vi "Line Configuration Dialog.vi"(8 "error in":errorcluster, 9 "engine configuration in":refnum<class "engine configuration.lvclass">, 10 "TDMS datalogger configuration":refnum<class "TDMS datalogger configuration.lvclass">, 11 "Line":T2) -> (0 "error out":errorcluster, 1 "success":bool, 2 "changed":bool, 3 "Mappings out":T1)   [LabVIEW 2015, in "TDMS datalogger editor node.lvclass"]
uses:
  TDMS datalogger editor node.lvclass
  <vilib>/NI/Module Execution Interface/Engine Configuration/engine configuration.lvclass
  <vilib>/NI/Tag Bus Module Framework/channel/TBM channel.lvclass
  module/configuration/TDMS datalogger configuration.lvclass
  <vilib>/NI/Tag Bus/tag/tag descriptor.lvclass/tag descriptor.ctl
  <vilib>/NI/Configuration Framework/serializable configuration/NISE_CEF_serializable configuration.lvclass/NISE_CEF_serializable configuration.ctl
  <vilib>/NI/Tag Bus/tag/write tag name.vi
  <vilib>/NI/Configuration Framework/serializable configuration/Read UID.vi
  <vilib>/NI/Tag Bus/tag/read data type.vi
  <vilib>/Utility/LVClass/Get LV Class Name.vi
  <vilib>/NI/Configuration Framework/error generator/NISE_error generator.vi
  <vilib>/NI/Tag Bus/tag/tag descriptor.lvclass
  <vilib>/NI/DCAF UI Toolkit/Controls/DCAF UI Elements.lvlib
panel:
  in  "Tag":i32(listbox)
  in  "Property Name":string
  in  "ok":bool
  in  "cancel":bool
  out "errors":string
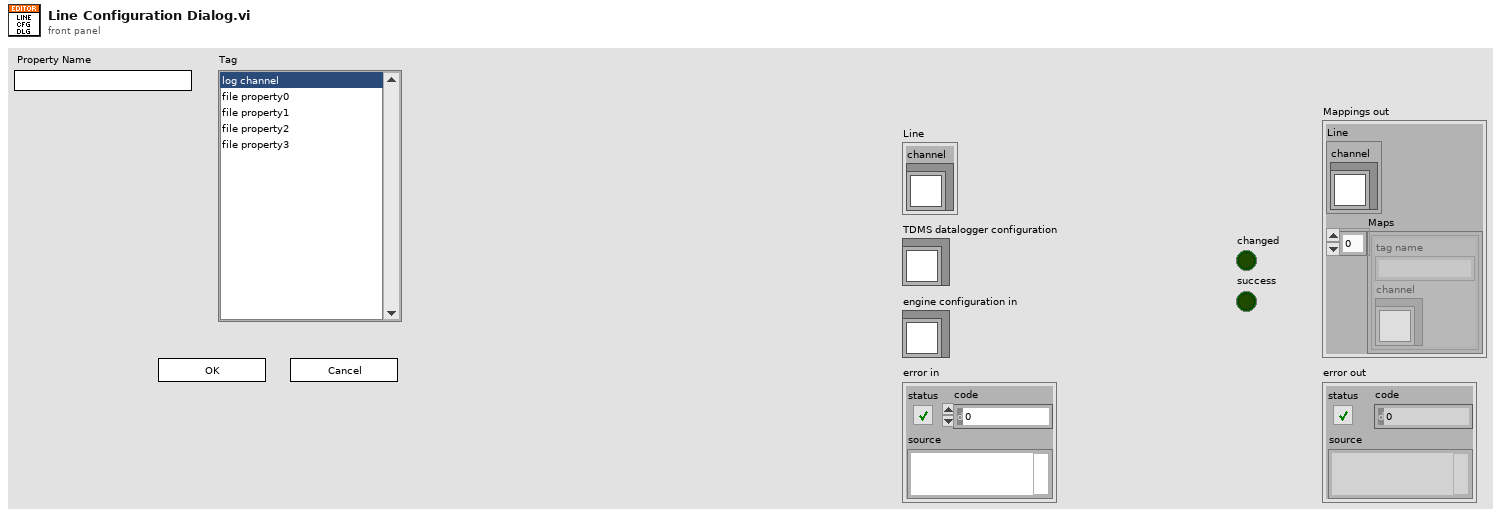
[diagram p1: front panel]
types:
  T1 = cluster{"Line":cluster{"channel":refnum<class "TBM channel.lvclass">}, "Maps":cluster{"tag name":string, "channel":refnum<class "TBM channel.lvclass">}[]}
  T2 = cluster{"channel":refnum<class "TBM channel.lvclass">}
  T3 = enum8{"Enabled", "Disabled", "Disabled and Grayed Out"}
  T4 = cluster{"tag name":string, "channel":refnum<class "TBM channel.lvclass">}
  T5 = cluster{"tag name":string, "channel":refnum<class "TBM channel.lvclass">}[]
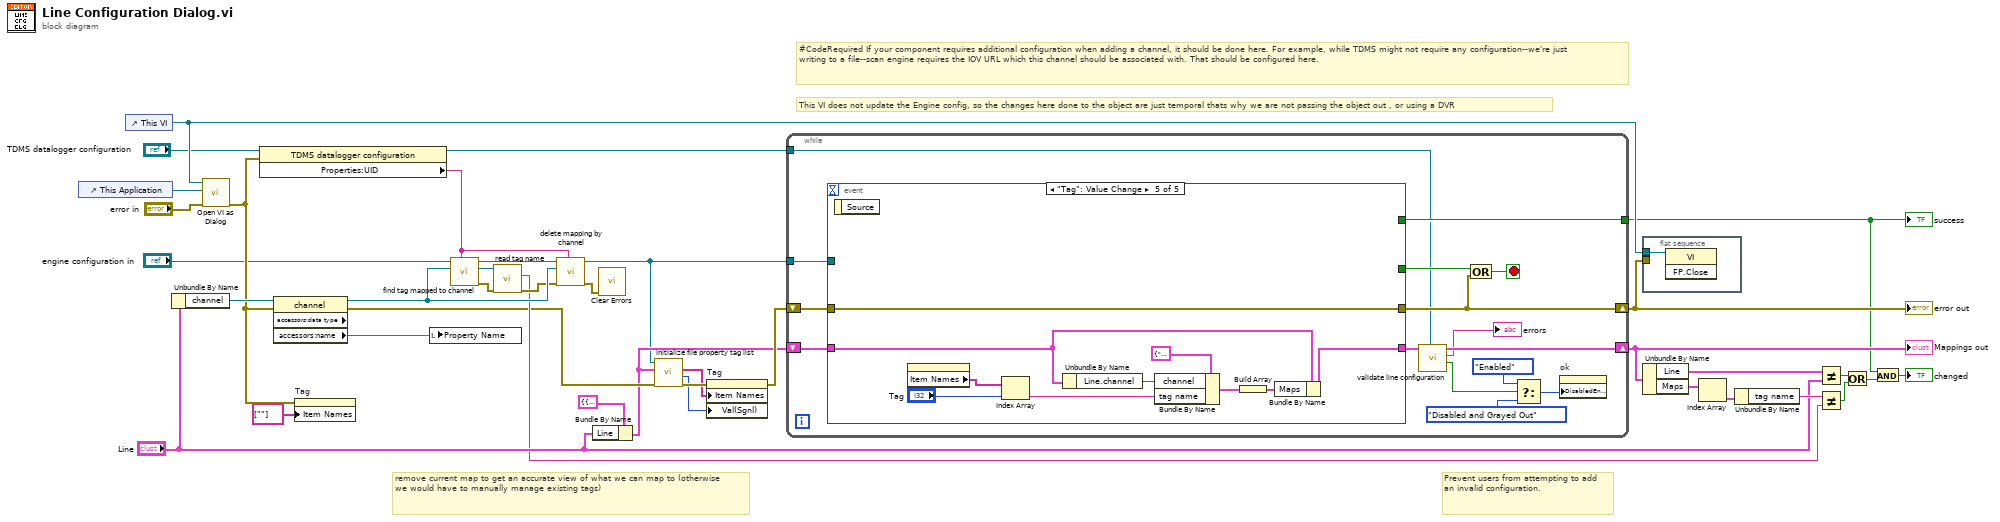
[diagram p0: block diagram]
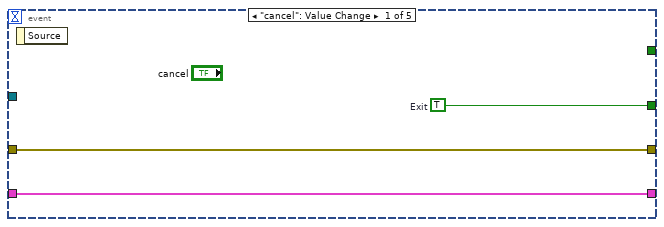
[diagram p2: hidden frame]
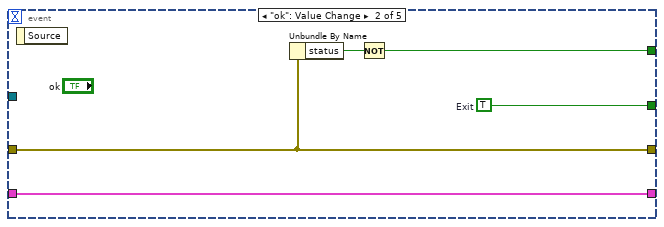
[diagram p3: hidden frame]
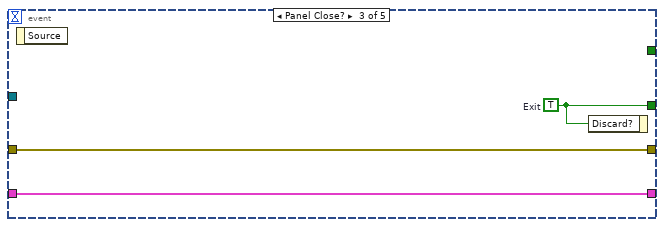
[diagram p4: hidden frame]
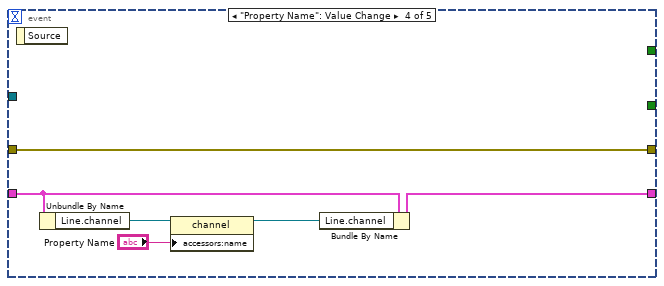
[diagram p5: hidden frame]
diagram:
  # "Prevent users from attempting to add an invalid configuration."
  # "This VI does not update the Engine config, so the changes here done to the object are just temporal thats why we are not passing the object out , or using a DVR"
  # "remove current map to get an accurate view of what we can map to (otherwise we would have to manually manage existing tags)"
  # "#CodeRequired If your component requires additional configuration when adding a channel, it should be done here. For example, while TDMS might not require any configuration--we're just writing to a file--scan engine requires the IOV URL which this channel should be associated with. That should be configured here."
  n1 = control-ref of="This Application"() -> (w33:refnum<vi>)
  n2 = control-ref of="This VI"() -> (w18:refnum<vi>)
  n3 = Unbundle By Name("Line") -> ("channel"=w38:refnum<class "TBM channel.lvclass">)
  n4 = call <vilib>:"Open VI as Dialog.vi"("error in (no error)"="error in", "This Application"=w33, "VI in"=w18) -> ("error out"=w31:errorcluster)  [unwired: 8 in]
  n5 = property class="TDMS datalogger configuration"(reference="TDMS datalogger configuration", error in=w31) -> (reference out=w28:refnum<class "TDMS datalogger configuration.lvclass">, "Properties:UID"=w17:string)  [unwired: 1 out]
  n6 = property class="channel" props=["accessors:data type", "accessors:name"](reference=w38, error in=w31) -> (reference out=w27:refnum<class "TBM channel.lvclass">, error out=w3:errorcluster, "accessors:name"=w16:string)  [unwired: 1 out]
  n7 = property on="Tag" class="LstBox (strict)"(error in=w31, "Item Names"=string[] [""]) -> ()  [unwired: 1 in, 2 out]
  n8 = local write "Property Name"(w16) -> ()
  n9 = call <vilib>:"find tag mapped to channel.vi"("owner"=w17, "channel"=w27, "engine configuration in"="engine configuration in") -> ("error out"=w25:errorcluster, "tag"=w26:refnum<class "tag descriptor.lvclass">, "engine configuration out"=w29:refnum<class "engine configuration.lvclass">)  [unwired: 6 in]
  n10 = call <vilib>:"read tag name.vi"("error in"=w25, "system tag in"=w26) -> ("error out"=w24:errorcluster, "name"=w8:string)  [unwired: 7 in, 1 out]
  n11 = call <vilib>:"delete mapping by channel.vi"("owner ID"=w17, "error in"=w24, "channel"=w27, "engine configuration in"=w29) -> ("error out"=w36:errorcluster, "engine configuration out"=w1:refnum<class "engine configuration.lvclass">)  [unwired: 6 in]
  n12 = Bundle By Name(cluster=T1 {"Line"={"channel"=refnum}, "Maps"=[]} ("Mappings"), "Line"="Line") -> (w2:T1)
  n13 = call <vilib>:"Clear Errors.vi"("error in (no error)"=w36) -> ()  [unwired: 5 in, 2 out]
  n14 = call "initialize file property tag list.vi"("error in"=w3, "Line"=w2, "engine configuration in"=w1) -> ("error out"=w7:errorcluster, "Value"=w5:i32, "Item Names"=w6:string[])  [unwired: 6 in]
  n15 = property on="Tag" class="LstBox (strict)"(error in=w7, "Item Names"=w6, "Val(Sgnl)"=w5) -> (error out=w4:errorcluster)  [unwired: 1 in, 1 out]
  n16 = while {
    shift-right: [w47] -> w15
    shift-left: w4 -> [w52]
    tunnel: [w51] -> w14
    shift-right: [w41] -> w34
    shift-left: w2 -> [w48]
    tunnel: w1 -> [w53]
    tunnel: w28 -> [w42]
    stop <- w49 stop-if-true
    n17 = event shown="[4] \"Tag\": Value Change" {
      selector: _ -> [_ _ _ _ _]
      dyn-events: _ -> [_ _ _ _ _]
      timeout: _ -> [_ _ _ _ _]
      tunnel: w53 -> [_ _ _ _ _]
      tunnel: w52 -> [w56 w59 w64 w70 w80]
      tunnel: [w56 w59 w64 w70 w80] -> w47
      tunnel: [_ w57 _ _ _] -> w51
      tunnel: [w54 w60 w62 _ _] -> w50
      tunnel: w48 -> [w55 w61 w63 w68 w72]
      tunnel: [w55 w61 w63 w69 w74] -> w43
      event "cancel": Value Change {
        w54 = TRUE  # Exit
        n18 = event-data() -> ()  [unwired: 1 in, 1 out]
      }
      event "ok": Value Change {
        w60 = TRUE  # Exit
        n19 = event-data() -> ()  [unwired: 1 in, 1 out]
        n20 = Unbundle By Name(w59) -> ("status"=w58:bool)
        n21 = Not(x=w58) -> (.not. x?=w57:bool)
      }
      event Panel Close? {
        w62 = TRUE  # Exit
        n22 = event-data() -> ()  [unwired: 1 in, 1 out]
        n23 = event-data("Discard?"=w62) -> ()  [unwired: 1 in, 1 out]
      }
      event "Property Name": Value Change {
        n24 = event-data() -> ()  [unwired: 1 in, 1 out]
        n25 = Unbundle By Name(w68) -> ("Line.channel"=w67:refnum<class "TBM channel.lvclass">)
        n26 = property class="channel"(reference=w67, "accessors:name"="Property Name") -> (reference out=w66:refnum<class "TBM channel.lvclass">)  [unwired: 1 in, 1 out]
        n27 = Bundle By Name(cluster=w68, "Line.channel"=w66) -> (w69:T1)
      }
      event "Tag": Value Change {
        n28 = event-data() -> ()  [unwired: 1 in, 1 out]
        n29 = property on="Tag" class="LstBox (strict)"() -> ("Item Names"=w78:string[])  [unwired: 2 in, 2 out]
        n30 = Index Array(array=w78, index="Tag") -> (element=w73:string)
        n31 = Unbundle By Name(w72) -> ("Line.channel"=w77:refnum<class "TBM channel.lvclass">)
        n32 = Bundle By Name(cluster=T4 {"tag name"="", "channel"=refnum} ("Cluster"), "channel"=w77, "tag name"=w73) -> (w76:T4)
        n33 = Build Array(w76) -> (w75:T5)
        n34 = Bundle By Name(cluster=w72, "Maps"=w75) -> (w74:T1)
      }
    }
    n35 = call "validate line configuration.vi"("TDMS datalogger configuration"=w42, "Mappings in"=w43) -> ("valid?"=w39:bool, "errors"=→"errors":string, "Mappings out"=w41:T1)  [unwired: 7 in]
    n36 = Compound Arithmetic op=OR(w50, w47) -> (w49:bool)
    n37 = Select(t=T3."Enabled" ("Disabled"), s=w39, f=T3."Disabled and Grayed Out") -> (s? t:f=w44:T3)
    n38 = property on="ok" class="Bool"("DisabledEnum"=w44) -> ()  [unwired: 2 in, 2 out]
  }
  "error out" <- w15
  "success" <- w14
  "Mappings out" <- w34
  n39 = flat-sequence {
    tunnel: w15 -> [_]
    tunnel: w18 -> [w81]
    frame #0 {
      n40 = invoke class="VI" method="FP.Close"(reference=w81) -> ()  [unwired: 2 in, 3 out]
    }
  }
  n41 = Unbundle By Name(w34) -> ("Line"=w35:T2, "Maps"=w23:T5)
  n42 = Index Array(array=w23) -> (element=w22:T4)  [unwired: 1 in]
  n43 = Unbundle By Name(w22) -> ("tag name"=w21:string)
  n44 = Not Equal?(x=w35, y="Line") -> (x != y?=w19:bool)
  n45 = Not Equal?(x=w21, y=w8) -> (x != y?=w20:bool)
  n46 = Or(x=w19, y=w20) -> (x .or. y?=w13:bool)
  n47 = And(x=w14, y=w13) -> (x .and. y?=→"changed":bool)
